vi "RTO.vi"(0 "System no.":i32=1 min=1 max=4 step=1, 2 "Affected axes":string[](array[string]), 3 "All axes?":bool, 4 "Axis identifier?":bool=TRUE, 5 "error in":errorcluster) -> (19 "error out":errorcluster)   [LabVIEW 2020]
doc: "Ready to turn off. The current position of the given axes is written to non-volatile memory, the servo is switched off automatically and RNP is performed to reduce the applied voltages to 0. When the controller is switched on next time, the saved position is read from non-volatile memory and set as current position. RTO can only be executed if the axis was referenced (e.g. with FNL, FPL, FRF or POS, etc.).\nRTO must be repeated when it was already performed in the current session but another motion occurred afterwards or the servo was switched on again.\n\nE-755: If All axes? = TRUE, then Axis identifier? can be FALSE. Command not available for E-755.101"
panel:
  # "Ready to turn off."
  # "If all axes: use"
  # "Halt"
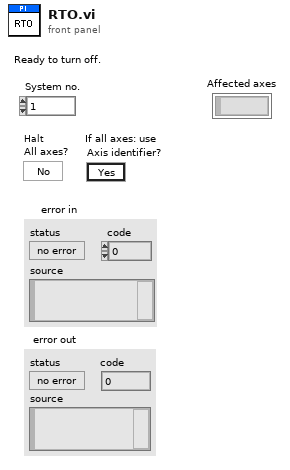
[diagram p1: front panel]
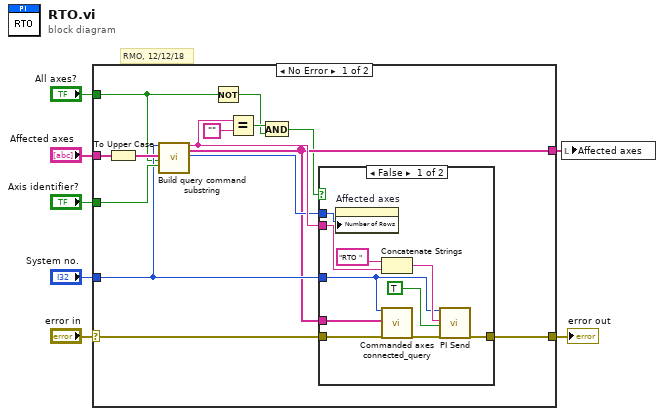
[diagram p0: block diagram]
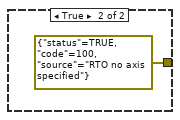
[diagram p2: hidden frame]
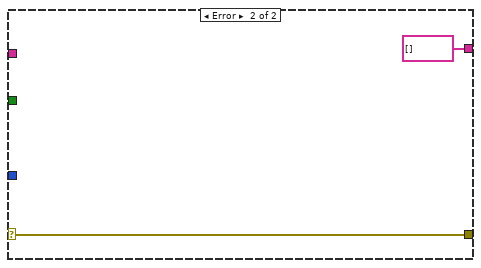
[diagram p3: hidden frame]
diagram:
  # "RMO, 12/12/18"
  n1 = case shown="No Error" "error in" {
    selector: "error in" -> [w10 w33]
    tunnel: "Affected axes" -> [w21 _]
    tunnel: [w9 w33] -> w6
    tunnel: "Axis identifier?" -> [w18 _]
    tunnel: "System no." -> [w15 _]
    tunnel: [w14 string[] [] ("Axes to query out")] -> w3
    tunnel: "All axes?" -> [w13 _]
    frame No Error {
      n2 = To Upper Case(1:w21) -> (0:w19:string[])
      n3 = call "Build query command substring.vi"("System no."=w15, "Axes to query in"=w19, "Query\nAll axes?"=w13, "For all axes: use\nAxis identifier?"=w18) -> ("Command substring"=w17:string, "Axes to query out"=w14:string[], "Number of rows"=w16:u32)  [unwired: 2 in, 11 out]
      n4 = Not(x=w13) -> (.not. x?=w11:bool)
      n5 = Equal?(x=w17, y="" ("x")) -> (x = y?=w12:bool)
      n6 = And(x=w12, y=w11) -> (x .and. y?=w8:bool)
      n7 = case shown="False" w8 {
        tunnel: w17 -> [w28 _]
        tunnel: w16 -> [w27 _]
        tunnel: w15 -> [w26 _]
        tunnel: w14 -> [w25 _]
        tunnel: w10 -> [w23 _]
        tunnel: [w22 errorcluster {"status"=TRUE, "code"=100, "source"="RTO no axis specified"} ("error out")] -> w9
        frame False {
          n8 = property on="Affected axes" class="Arr (strict)"("Number of Rows"=w27) -> ()  [unwired: 2 in, 2 out]
          n9 = Concatenate Strings("RTO ", w28) -> (w29:string)
          n10 = call "Commanded axes connected_query.vi"("System no."=w26, "Commanded axes"=w25, "error in"=w23) -> ("error out"=w24:errorcluster)  [unwired: 1 in, 15 out]
          n11 = call "PI Send.vi"("System no."=w26, "String to send"=w29, "Attach termination char.?"=TRUE ("Attach Linefeed?"), "error in"=w24) -> ("error out"=w22:errorcluster)  [unwired: 2 in, 13 out]
        }
        frame True {
        }
      }
    }
    frame Error {
    }
  }
  "error out" <- w6
  n12 = local write "Affected axes"(w3) -> ()
